vi "坐标平移(标量）.vi"(8 "Error In":errorcluster caption="错误输入", 9 "dy":dbl, 10 "dx":dbl, 11 "输入点":T1 caption="点（双精度）") -> (0 "Error Out":errorcluster caption="错误输出", 3 "输出点":T1 caption="点（双精度）")   [LabVIEW 2012, in "几何工具.lvlib"]
uses:
  <vilib>/Utility/miscctls.llb/LVPointDoubleTypeDef.ctl
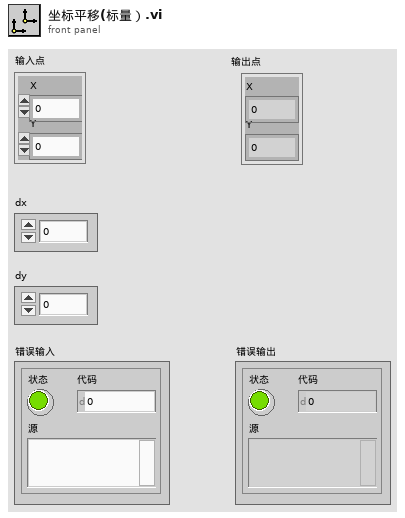
[diagram p1: front panel]
types:
  T1 = typedef "LVPointDoubleTypeDef.ctl" = cluster{"X":dbl, "Y":dbl}
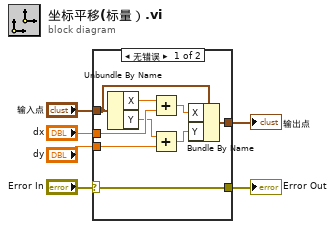
[diagram p0: block diagram]
diagram:
  n1 = case shown="无错误" "Error In" {
    selector: "Error In" -> [w15 w17]
    tunnel: [w15 w17] -> w5
    tunnel: "输入点" -> [w10 w16]
    tunnel: "dx" -> [w13 _]
    tunnel: "dy" -> [w11 _]
    tunnel: [w7 w16] -> w1
    frame No Error {
      n2 = Unbundle By Name(w10) -> ("X"=w14:dbl, "Y"=w12:dbl)
      n3 = Add(x=w14, y=w13) -> (x+y=w9:dbl)
      n4 = Add(x=w12, y=w11) -> (x+y=w8:dbl)
      n5 = Bundle By Name(cluster=w10, "X"=w9, "Y"=w8) -> (w7:T1)
    }
    frame Error {
    }
  }
  "Error Out" <- w5
  "输出点" <- w1
